vi "GetEncoderDistance.vi"(8 "Error In":errorcluster, 11 "Distance":dbl) -> (0 "Error Out":errorcluster, 3 "Distance Travelled (in)":dbl)   [LabVIEW 2017]
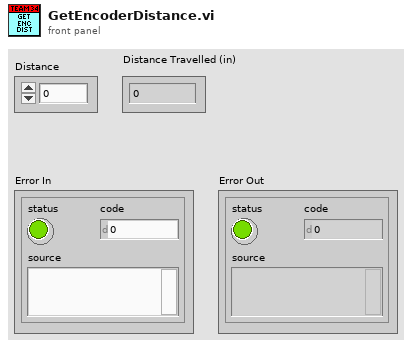
[diagram p1: front panel]
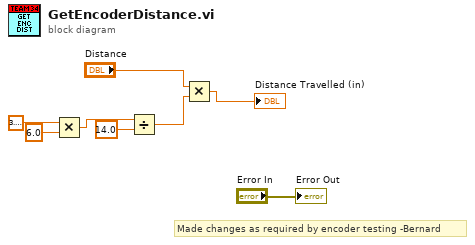
[diagram p0: block diagram]
diagram:
  # "Made changes as required by encoder testing -Bernard"
  n1 = Multiply(x=3.141592653589793, y=6.0) -> (x*y=w3:dbl)
  n2 = Divide(x=w3, y=14.0) -> (x/y=w1:dbl)
  n3 = Multiply(x="Distance", y=w1) -> (x*y=→"Distance Travelled (in)":dbl)
  "Error Out" <- "Error In"
